vi "test Tx Duration.vi"(8 "error in (no error)":errorcluster, 11 "TestCase in":refnum<class "Performance Tests.lvclass">=refnum) -> (0 "error out":errorcluster, 3 "TestCase out":refnum<class "Performance Tests.lvclass">)   [LabVIEW 2021, in "Performance Tests.lvclass"]
uses:
  Performance Tests.lvclass
  Classes/Performance/Performance.lvclass
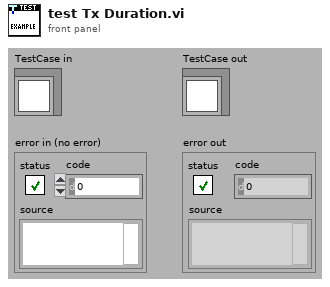
[diagram p1: front panel]
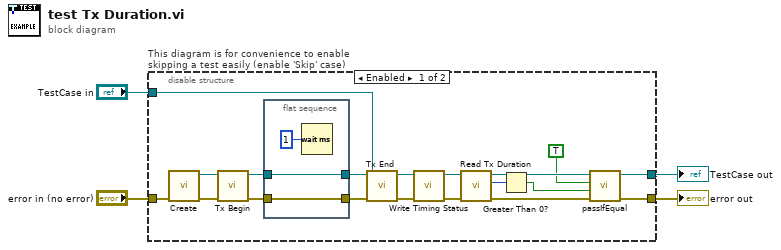
[diagram p0: block diagram]
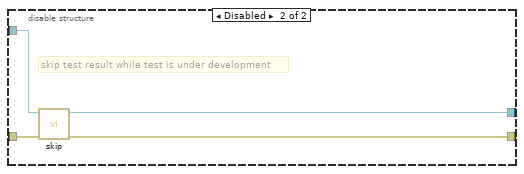
[diagram p2: hidden frame]
diagram:
  n1 = disable-structure "This diagram is for convenience to enable skipping a test easily (enable 'Skip' case)" shown="Enabled" {
    disable-tunnel: "TestCase in" -> [w21 w29]
    disable-tunnel: [w20 w27] -> w1
    disable-tunnel: [w22 w28] -> w3
    disable-tunnel: "error in (no error)" -> [w8 w26]
    frame Enabled {
      n2 = call "Create.vi"("error in (no error)"=w8) -> ("error out"=w19:errorcluster, "performance"=w18:refnum<class "Performance.lvclass">)  [unwired: 9 in]
      n3 = call "Tx Begin.vi"("error in (no error)"=w19, "Performance in"=w18) -> ("error out"=w17:errorcluster, "Performance out"=w16:refnum<class "Performance.lvclass">)  [unwired: 8 in]
      n4 = flat-sequence {
        tunnel: w17 -> [w24]
        tunnel: w16 -> [w25]
        tunnel: [w25] -> w15
        tunnel: [w24] -> w14
        frame #0 {
          n5 = Wait (ms)(milliseconds to wait=u32 1) -> ()  [unwired: 1 out]
        }
      }
      n6 = call "Tx End.vi"("error in"=w14, "performance in"=w15) -> ("error out"=w11:errorcluster, "performance out"=w12:refnum<class "Performance.lvclass">)  [unwired: 8 in]
      n7 = call "Write Timing Status.vi"("error in"=w11, "framework performance in"=w12) -> ("error out"=w9:errorcluster, "framework performance out"=w10:refnum<class "Performance.lvclass">)  [unwired: 8 in]
      n8 = call "Read Tx Duration.vi"("error in (no error)"=w9, "Framework Performance in"=w10) -> ("error out"=w7:errorcluster, "tx duration"=w13:u32)  [unwired: 7 in, 1 out]
      n9 = Greater Than 0?(x=w13) -> (x > 0?=w6:bool)
      n10 = call-dynamic "passIfEqual.vi"("error in (no error)"=w7, "y"=w6, "x"=TRUE, "TestCase in"=w21) -> ("error out"=w22:errorcluster, "TestCase out"=w20:refnum<class "Performance Tests.lvclass">)  [unwired: 6 in]
    }
    frame Disabled {
      # "skip test result while test is under development"
      n11 = call <vilib>:"skip.vi"("error in (no error)"=w26, "TestCase in"=w29) -> ("error out"=w28:errorcluster, "TestCase out"=w27:refnum<class "Performance Tests.lvclass">)  [unwired: 8 in]
    }
  }
  "error out" <- w3
  "TestCase out" <- w1
